vi "1 SiO2 Material Properties GAP.vi"(6 "NS Base Area":dbl, 8 "Sio2 Thickness 2":dbl, 11 "Energy (Heat; I^2R)":dbl) -> (1 "SiO2 Specfic Heat Capacity":dbl, 2 "Mass SiO2":dbl, 3 "SilO2 Density":dbl, 4 "Delta Temp Change SiO2":dbl, 5 "Volume SiO2":dbl, 7 "Sio2 Thickness":dbl)   [LabVIEW 2020]
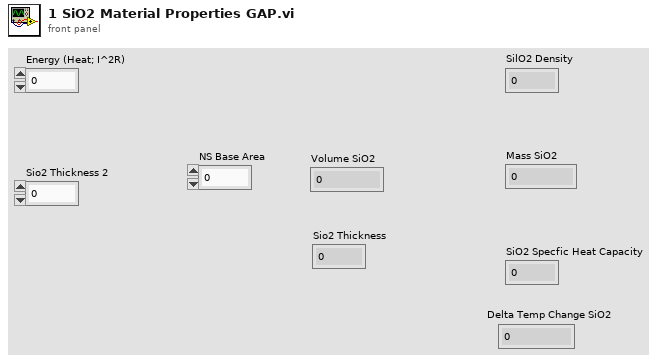
[diagram p1: front panel]
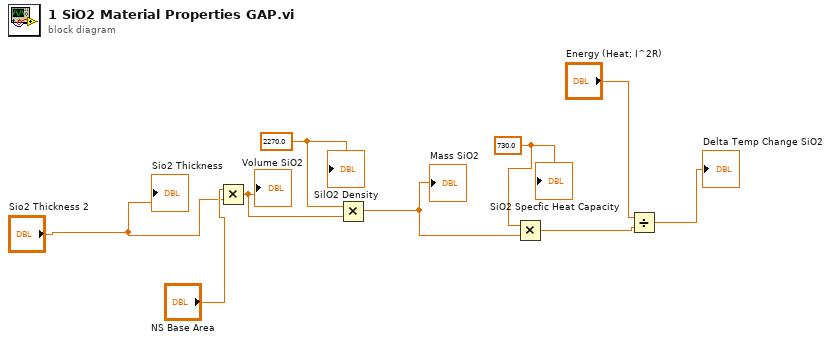
[diagram p0: block diagram]
diagram:
  w4 = 730.0 ("Silicon Specfic Heat Capacity 2")
  w2 = 2270.0 ("Silicon Dioxide Density 2")
  n1 = Multiply(x="NS Base Area", y="Sio2 Thickness 2") -> (x*y=w3:dbl)
  "Volume SiO2" <- w3
  n2 = Multiply(x=w2, y=w3) -> (x*y=w5:dbl)
  "Mass SiO2" <- w5
  n3 = Multiply(x=w4, y=w5) -> (x*y=w7:dbl)
  n4 = Divide(x="Energy (Heat; I^2R)", y=w7) -> (x/y=→"Delta Temp Change SiO2":dbl)
  "Sio2 Thickness" <- "Sio2 Thickness 2"
  "SilO2 Density" <- w2
  "SiO2 Specfic Heat Capacity" <- w4
